vi "I64.vi"(8 "error in (no error)":errorcluster, 10 "Timeout":i32=-1, 11 "Notifier in":refnum<class "Notifier.lvclass">=refnum) -> (0 "error out":errorcluster, 1 "Timeout?":bool, 2 "Notification Out":i64=-1, 3 "Notifier out":refnum<class "Notifier.lvclass">)   [LabVIEW 2019]
uses:
  Notifier.lvclass
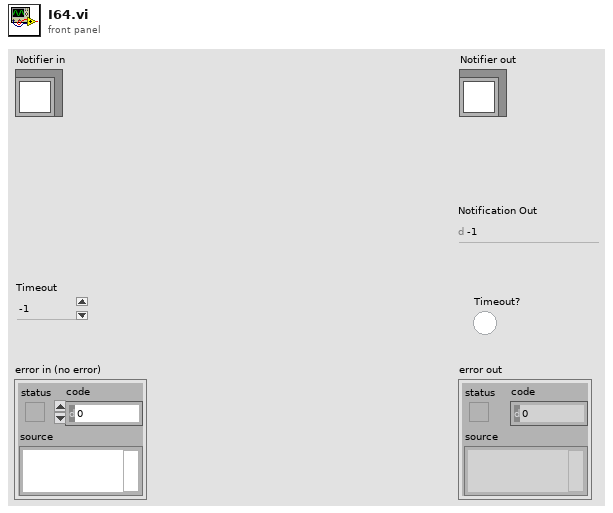
[diagram p1: front panel]
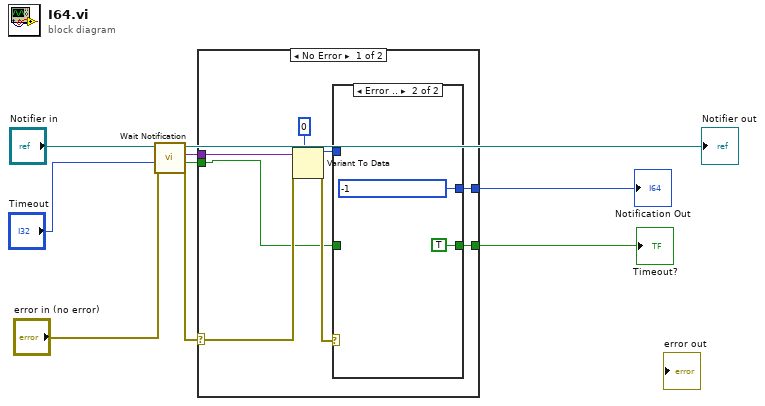
[diagram p0: block diagram]
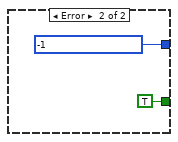
[diagram p3: hidden frame]
diagram:
  n1 = call-dynamic "Wait Notification.vi"("error in (no error)"="error in (no error)", "Timeout"="Timeout", "Notifier in"="Notifier in") -> ("error out"=w6:errorcluster, "Timeout?"=w5:bool, "Notification"=w4:variant, "Notifier out"=→"Notifier out":refnum<class "Notifier.lvclass">)  [unwired: 5 in]
  n2 = case shown="No Error" w6 {
    selector: w6 -> [w15 _]
    tunnel: w5 -> [w12 _]
    tunnel: w4 -> [w17 _]
    tunnel: [w11 TRUE ("Timeout?")] -> w2
    tunnel: [w10 i64 -1] -> w1
    frame No Error {
      n3 = Variant To Data(error in=w15, type=i64 0, Variant=w17) -> (data=w13:i64, error out=w14:errorcluster)
      n4 = case shown="Error .." w14 {
        tunnel: w12 -> [w19 _]
        tunnel: [w19 TRUE ("Timeout?")] -> w11
        tunnel: w13 -> [w18 _]
        tunnel: [w18 i64 -1] -> w10
        frame No Error {
        }
        frame Error {
        }
      }
    }
    frame Error {
    }
  }
  "Timeout?" <- w2
  "Notification Out" <- w1
